vi "SelectedMotionProfileMode.vi"() -> ()   [LabVIEW 2017]
panel:
  in  "Reset":bool
  in  "Forward":i16
  in  "End Heading":dbl
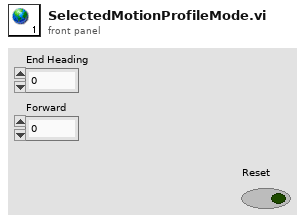
[diagram p1: front panel]
diagram:
